vi "Sub-falling edge.vi"(0 "LS1_DI":bool, 5 "LS2_DI":bool, 7 "LS3_DI":bool, 9 "LS4_DI":bool, 11 "LS5_DI":bool) -> (1 "LS1_Shift":bool, 2 "LS2_Shift":bool, 3 "LS3_Shift":bool, 4 "LS1_DO":bool, 6 "LS2_DO":bool, 8 "LS3_DO":bool, 10 "LS4_DO":bool, 13 "LS4_Shift":bool, 14 "LS5_Shift":bool, 15 "LS5_DO":bool)   [LabVIEW 2017]
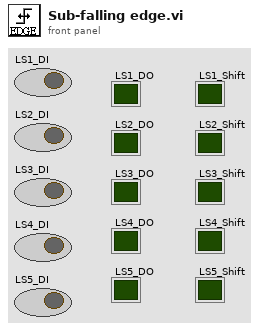
[diagram p1: front panel]
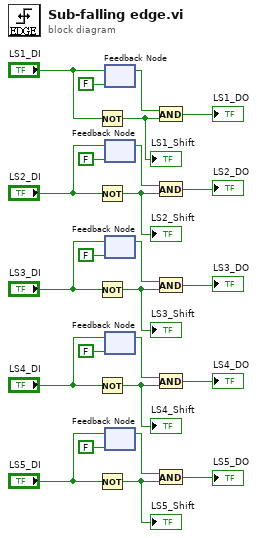
[diagram p0: block diagram]
diagram:
  n1 = Not(x="LS1_DI") -> (.not. x?=w22:bool)
  "LS1_Shift" <- w22
  n2 = Not(x="LS2_DI") -> (.not. x?=w6:bool)
  "LS2_Shift" <- w6
  n3 = Not(x="LS3_DI") -> (.not. x?=w10:bool)
  "LS3_Shift" <- w10
  n4 = Not(x="LS4_DI") -> (.not. x?=w14:bool)
  "LS4_Shift" <- w14
  n5 = Not(x="LS5_DI") -> (.not. x?=w21:bool)
  "LS5_Shift" <- w21
  n6 = feedback #1(FALSE ("DI Value")) -> (w24:bool)
  n7 = feedback-in #1("LS1_DI") -> ()
  n8 = feedback #2(FALSE ("DI Value")) -> (w8:bool)
  n9 = feedback-in #2("LS2_DI") -> ()
  n10 = feedback #3(FALSE ("DI Value")) -> (w12:bool)
  n11 = feedback-in #3("LS3_DI") -> ()
  n12 = feedback #4(FALSE ("DI Value")) -> (w16:bool)
  n13 = feedback-in #4("LS4_DI") -> ()
  n14 = feedback #5(FALSE ("DI Value")) -> (w19:bool)
  n15 = feedback-in #5("LS5_DI") -> ()
  n16 = And(x=w24, y=w22) -> (x .and. y?=→"LS1_DO":bool)
  n17 = And(x=w8, y=w6) -> (x .and. y?=→"LS2_DO":bool)
  n18 = And(x=w12, y=w10) -> (x .and. y?=→"LS3_DO":bool)
  n19 = And(x=w16, y=w14) -> (x .and. y?=→"LS4_DO":bool)
  n20 = And(x=w19, y=w21) -> (x .and. y?=→"LS5_DO":bool)
